vi "Run Action_Do.vi"(8 "error in (no error)":errorcluster, 11 "Set Version from Git Tag":refnum<class "Set Version from Git Tag.lvclass">) -> (0 "error out":errorcluster, 1 "Success?":bool, 3 "Report Array":refnum<class "Report Data.lvclass">[](array[class]))   [LabVIEW 2020, in "ProjectBuilder.lvlib" / "Set Version from Git Tag.lvclass"]
uses:
  Set Version from Git Tag.lvclass
  Action/Project Action/Project Action.lvclass
  ProjectBuilder.lvlib
  <vilib>/AppBuilder/AB_API_Simple/Build Specification Version.ctl
  <vilib>/AppBuilder/AB_API_Simple/NI_App_Builder_API.lvlib
  Version Data/Version Data.lvclass
  C:/Current projects/WS/LV32.2020..ProjectBuilder/Class/Action/Project Action/Project Action.lvclass
  C:/Current projects/WS/LV32.2020..ProjectBuilder/Interface/Project Action Interface/Project Action Interface.lvclass
  C:/Current projects/WS/LV32.2020..ProjectBuilder/Class/Set Version from Git Tag/Set Version from Git Tag.lvclass
  C:/Current projects/WS/LV32.2020..ProjectBuilder/Class/Data/Report Data/Report Data.lvclass
  C:/Current projects/WS/LV32.2020..ProjectBuilder/Class/Set Version from Git Tag/Version Data/Version Data.lvclass
  Data/Report Data/Report Data.lvclass
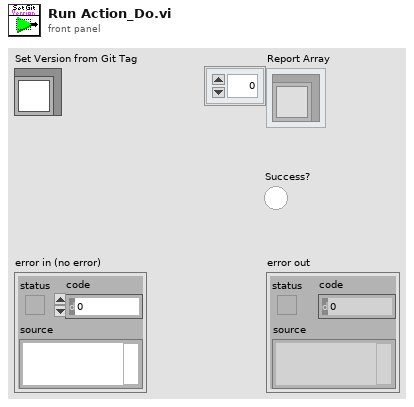
[diagram p1: front panel]
types:
  T1 = typedef "NI_App_Builder_API.lvlib/Build Specification Version.ctl" = cluster{"Major":u16, "Minor":u16, "Fix":u16, "Build":u16}
  T2 = cluster{"Build Specification Version[0]":i32, "Build Specification Version[1]":i32, "Build Specification Version[2]":i32, "Build Specification Version[3]":i32}
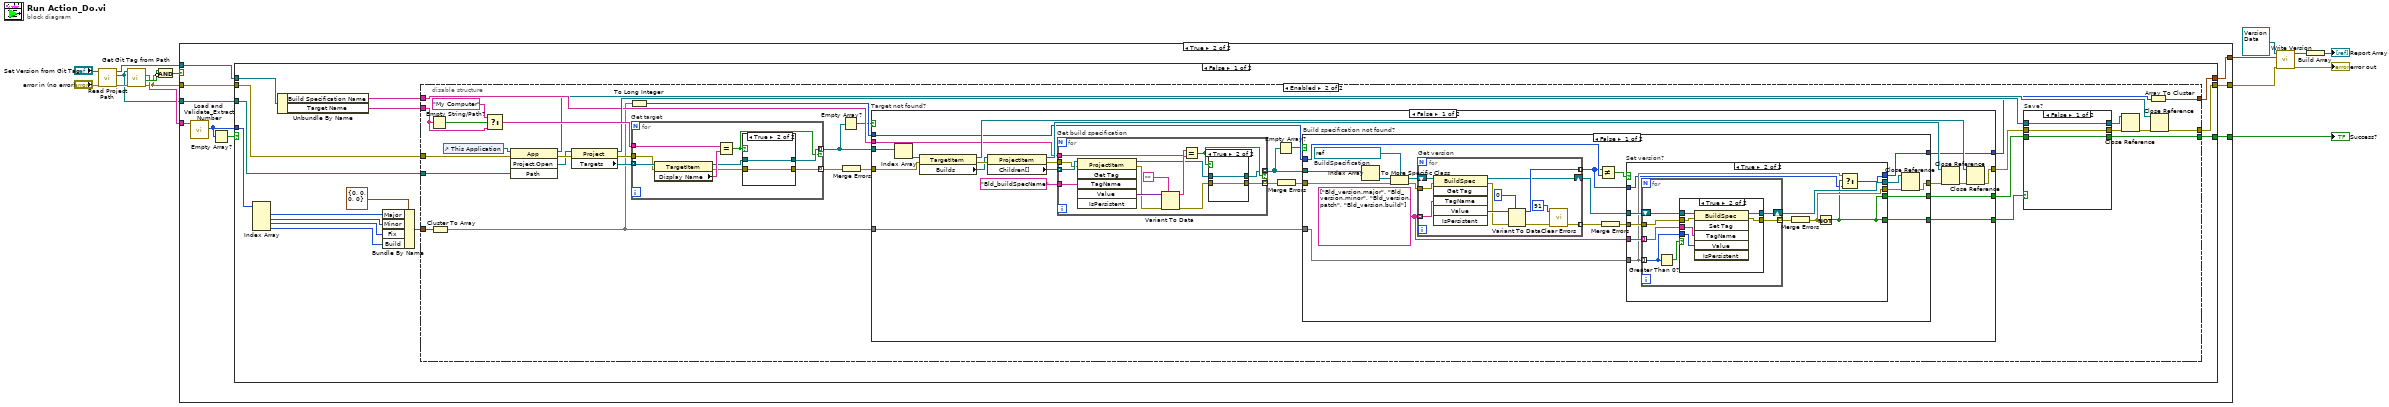
[diagram p0: block diagram]
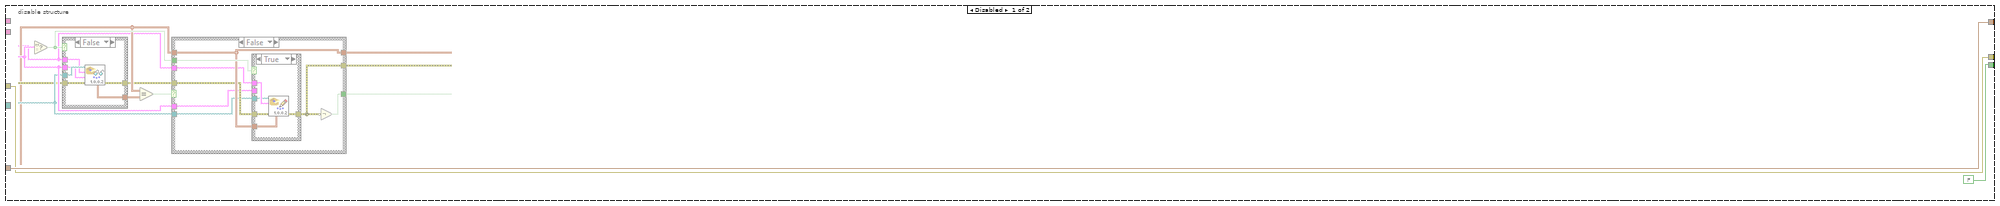
[diagram p3: hidden frame]
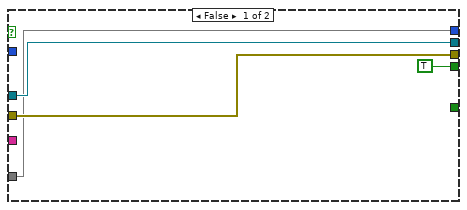
[diagram p4: hidden frame]
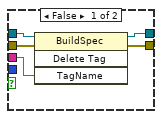
[diagram p5: hidden frame]
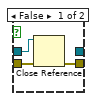
[diagram p7: hidden frame]
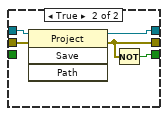
[diagram p9: hidden frame]
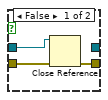
[diagram p10: hidden frame]
diagram:
  n1 = call "Read Project Path.vi"("error in (no error)"="error in (no error)", "Project Action in"="Set Version from Git Tag") -> ("error out"=w14:errorcluster, "Project Path"=w10:path, "Project Action out"=w8:refnum<class "Set Version from Git Tag.lvclass">)  [unwired: 7 in]
  n2 = call "Get Git Tag from Path.vi"("error in (no error)"=w14, "Path"=w10) -> ("error out"=w9:errorcluster, "Success?"=w13:bool, "Tag"=w11:string)  [unwired: 6 in, 1 out]
  n3 = Compound Arithmetic op=AND(w13, invert w9) -> (w12:bool)
  n4 = case shown="True" w12 {
    selector: w12 -> [w17 _]
    tunnel: w11 -> [_ w27]
    tunnel: w10 -> [_ w26]
    tunnel: [w18 w23] -> w7
    tunnel: w9 -> [w18 w24]
    tunnel: [w17 w22] -> w6
    tunnel: w8 -> [_ w25]
    tunnel: [_ w19] -> w1
    frame False {
    }
    frame True {
      n5 = call "Load and Validate_Extract Number.vi"("String"=w27) -> ("Number Array"=w21:i32[])  [unwired: 9 in, 1 out]
      n6 = Empty Array?(array=w21) -> (empty?=w20:bool)
      n7 = case shown="False" w20 {
        tunnel: w26 -> [w29 _]
        tunnel: w25 -> [w37 _]
        tunnel: w24 -> [w30 w205]
        tunnel: [w28 w205] -> w23
        tunnel: [w36 _] -> w22
        tunnel: w21 -> [w35 _]
        tunnel: [w32 _] -> w19
        frame False {
          n8 = Index Array(array=w35) -> (element #1=w41:i32, element #2=w40:i32, element #3=w39:i32, element #4=w38:i32)  [unwired: 4 in]
          n9 = Unbundle By Name(w37) -> ("Build Specification Name"=w34:string, "Target Name"=w31:string)
          n10 = Bundle By Name(cluster=T1 {"Major"=0, "Minor"=0, "Fix"=0, "Build"=0} ("Build Specification Version"), "Major"=w41, "Minor"=w40, "Fix"=w39, "Build"=w38) -> (w33:T1)
          n11 = disable-structure shown="Enabled" {
            disable-tunnel: [FALSE w51] -> w36
            disable-tunnel: w34 -> [_ w62]
            disable-tunnel: w33 -> [w45 w61]
            disable-tunnel: [w45 w48] -> w32
            disable-tunnel: w31 -> [_ w63]
            disable-tunnel: w30 -> [w44 w57]
            disable-tunnel: w29 -> [_ w56]
            disable-tunnel: [w44 w53] -> w28
            frame Disabled {
            }
            frame Enabled {
              n12 = Empty String/Path?(string/path=w63) -> (empty?=w71:bool)
              n13 = Cluster To Array(cluster=w61) -> (array=w60:u16[])
              n14 = control-ref of="This Application"() -> (w55:refnum<vi>)
              n15 = Select(t="My Computer", s=w71, f=w63) -> (s? t:f=w72:string)
              n16 = invoke class="App" method="Project.Open"(reference=w55, error in=w57, "Path"=w56) -> (reference out=w52:refnum<vi>, error out=w70:errorcluster, "Project:Open"=w65:refnum<vi>)  [unwired: 1 in, 1 out]
              n17 = property class="Project"(reference=w65, error in=w70) -> (reference out=w67:refnum<vi>, error out=w75:errorcluster, "Targets"=w73:refnum<vi>[])
              n18 = To Long Integer(number=w60) -> (32bit integer=w59:i32[])
              n19 = for "Get target" {
                tunnel: w73 -> [w199] mode=indexing
                tunnel: w72 -> [w197]
                tunnel: [w195] -> w47 mode=indexing if=w191
                tunnel: w75 -> [w194]
                tunnel: [w192] -> w74 mode=indexing
                n20 = property class="TargetItem"(reference=w199, error in=w194) -> (reference out=w196:refnum<vi>, error out=w193:errorcluster, "Display Name"=w198:string)
                n21 = Equal?(x=w197, y=w198) -> (x = y?=w191:bool)
                n22 = case shown="True" w191 {
                  tunnel: [_ w204] -> w195
                  tunnel: w196 -> [w202 w204]
                  tunnel: w193 -> [w201 w203]
                  tunnel: [w200 w203] -> w192
                  frame False {
                    n23 = Close Reference(reference=w202, error in (no error)=w201) -> (error out=w200:errorcluster)
                  }
                  frame True {
                  }
                }
              }
              n24 = Empty Array?(array=w47) -> (empty?=w46:bool)
              n25 = Merge Errors(w74) -> (w76:errorcluster)
              n26 = case "Target not found?" shown="False" w46 {
                tunnel: w76 -> [w99 w182]
                tunnel: w47 -> [w97 _]
                tunnel: [w91 w182] -> w66
                tunnel: w62 -> [w84 _]
                tunnel: w60 -> [w83 _]
                tunnel: w59 -> [w82 _]
                tunnel: [w81 _] -> w58
                tunnel: [w80 _] -> w50
                tunnel: [w79 _] -> w49
                frame False {
                  n27 = Index Array(array=w97) -> (element=w86:refnum<vi>)  [unwired: 1 in]
                  n28 = property class="TargetItem"(reference=w86, error in=w99) -> (reference out=w98:refnum<vi>, error out=w92:errorcluster, "Builds"=w87:refnum<vi>)
                  n29 = property class="ProjectItem"(reference=w87, error in=w92) -> (reference out=w90:refnum<vi>, error out=w95:errorcluster, "Children[]"=w93:refnum<vi>[])
                  n30 = for "Get build specification" {
                    tunnel: w93 -> [w176] mode=indexing
                    tunnel: "Bld_buildSpecName" ("String") -> [w175]
                    tunnel: w84 -> [w171]
                    tunnel: w95 -> [w170]
                    tunnel: [w167] -> w78 mode=indexing if=w169
                    tunnel: [w164] -> w94 mode=indexing
                    n31 = invoke class="ProjectItem" method="Get Tag"(reference=w176, error in=w170, "TagName"=w175) -> (reference out=w168:refnum<vi>, error out=w166:errorcluster, "Value"=w174:variant)  [unwired: 3 in, 3 out]
                    n32 = Variant To Data(error in=w166, type="", Variant=w174) -> (data=w172:string, error out=w165:errorcluster)
                    n33 = Equal?(x=w171, y=w172) -> (x = y?=w169:bool)
                    n34 = case shown="True" w169 {
                      tunnel: [_ w181] -> w167
                      tunnel: w168 -> [w179 w181]
                      tunnel: w165 -> [w178 w180]
                      tunnel: [w177 w180] -> w164
                      frame False {
                        n35 = Close Reference(reference=w179, error in (no error)=w178) -> (error out=w177:errorcluster)
                      }
                      frame True {
                      }
                    }
                  }
                  n36 = Empty Array?(array=w78) -> (empty?=w77:bool)
                  n37 = Merge Errors(w94) -> (w96:errorcluster)
                  n38 = case "Build specification not found?" shown="False" w77 {
                    tunnel: w96 -> [w118 w163]
                    tunnel: w78 -> [w117 _]
                    tunnel: [w111 w163] -> w88
                    tunnel: w83 -> [w106 _]
                    tunnel: w82 -> [w104 _]
                    tunnel: [w103 _] -> w81
                    tunnel: [w102 _] -> w80
                    tunnel: [w100 _] -> w79
                    frame False {
                      w108 = string[] ["Bld_version.major", "Bld_version.minor", "Bld_version.patch", "Bld_version.build"]
                      w107 = refnum<vi> refnum  # BuildSpecification
                      n39 = Index Array(array=w117) -> (element=w109:refnum<vi>)  [unwired: 1 in]
                      n40 = To More Specific Class(target class=w107, reference=w109, error in=w118) -> (specific class reference=w116:refnum<vi>, error out=w115:errorcluster)
                      n41 = for "Get version" {
                        tunnel: w108 -> [w161] mode=indexing
                        tunnel: [w158] -> w101 mode=indexing
                        shift-right: [w157] -> w110
                        shift-left: w116 -> [w162]
                        tunnel: [w153] -> w113 mode=indexing
                        tunnel: w115 -> [w154]
                        n42 = invoke class="BuildSpec" method="Get Tag"(reference=w162, error in=w154, "TagName"=w161) -> (reference out=w157:refnum<vi>, error out=w156:errorcluster, "Value"=w160:variant)  [unwired: 3 in, 3 out]
                        n43 = Variant To Data(error in=w156, type=0, Variant=w160) -> (data=w158:i32, error out=w155:errorcluster)
                        n44 = call <vilib>:"Clear Errors.vi"("error in (no error)"=w155, "specific error code to clear (0: all)"=91) -> ("error out"=w153:errorcluster)  [unwired: 4 in, 1 out]
                      }
                      n45 = Not Equal?(x=w101, y=w104) -> (x != y?=w105:bool)
                      n46 = Merge Errors(w113) -> (w114:errorcluster)
                      n47 = case "Set version?" shown="True" w105 {
                        tunnel: [w123 w133] -> w119
                        tunnel: w114 -> [w122 w132]
                        tunnel: [w122 w128] -> w112
                        tunnel: w110 -> [w123 w130]
                        tunnel: w108 -> [_ w129]
                        tunnel: w106 -> [w120 w126]
                        tunnel: [_ w127] -> w103
                        tunnel: [TRUE w127] -> w102
                        tunnel: w101 -> [_ w125]
                        tunnel: [w120 w124] -> w100
                        frame False {
                        }
                        frame True {
                          n48 = for {
                            tunnel: w129 -> [w139] mode=indexing
                            shift-right: [w138] -> w133
                            shift-left: w130 -> [w140]
                            tunnel: w126 -> [w135] mode=indexing
                            tunnel: [w137] -> w131 mode=indexing
                            tunnel: w132 -> [w136]
                            n49 = Greater Than 0?(x=w135) -> (x > 0?=w134:bool)
                            n50 = case shown="True" w134 {
                              tunnel: w140 -> [w145 w151]
                              tunnel: w139 -> [w144 w150]
                              tunnel: [w143 w149] -> w138
                              tunnel: [w141 w148] -> w137
                              tunnel: w136 -> [w142 w147]
                              tunnel: w135 -> [_ w146]
                              frame False {
                                n51 = invoke class="BuildSpec" method="Delete Tag"(reference=w145, error in=w142, "TagName"=w144) -> (reference out=w143:refnum<vi>, error out=w141:errorcluster)  [unwired: 1 in, 2 out]
                              }
                              frame True {
                                n52 = invoke class="BuildSpec" method="Set Tag"(reference=w151, error in=w147, "TagName"=w150, "Value"=w146) -> (reference out=w149:refnum<vi>, error out=w148:errorcluster)  [unwired: 2 in, 4 out]
                              }
                            }
                          }
                          n53 = Merge Errors(w131) -> (w128:errorcluster)
                          n54 = Not(x=w128) -> (.not. x?=w127:bool)
                          n55 = Select(t=w126, s=w127, f=w125) -> (s? t:f=w124:i32[])
                        }
                      }
                      n56 = Close Reference(reference=w119, error in (no error)=w112) -> (error out=w111:errorcluster)
                    }
                    frame True {
                    }
                  }
                  n57 = Close Reference(reference=w90, error in (no error)=w88) -> (error out=w89:errorcluster)
                  n58 = Close Reference(reference=w98, error in (no error)=w89) -> (error out=w91:errorcluster)
                }
                frame True {
                }
              }
              n59 = case "Save?" shown="False" w58 {
                tunnel: [w184 w186] -> w69
                tunnel: [w185 w190] -> w68
                tunnel: w67 -> [w185 w189]
                tunnel: w66 -> [w184 w188]
                tunnel: [w183 w187] -> w51
                tunnel: w50 -> [w183 _]
                frame False {
                }
                frame True {
                  n60 = invoke class="Project" method="Save"(reference=w189, error in=w188) -> (reference out=w190:refnum<vi>, error out=w186:errorcluster)  [unwired: 2 in, 2 out]
                  n61 = Not(x=w186) -> (.not. x?=w187:bool)
                }
              }
              n62 = Close Reference(reference=w68, error in (no error)=w69) -> (error out=w54:errorcluster)
              n63 = Array To Cluster(array=w49) -> (cluster=w48:T2)
              n64 = Close Reference(reference=w52, error in (no error)=w54) -> (error out=w53:errorcluster)
            }
          }
        }
        frame True {
        }
      }
    }
  }
  "Success?" <- w6
  n65 = call "Write Version.vi"("error in (no error)"=w7, "Build Specification Version"=w1, "Version Data in"=refnum<class "Version Data.lvclass"> refnum ("ProjectBuilder.lvlib:Version Data.lvclass")) -> ("error out"=→"error out":errorcluster, "Version Data out"=w2:refnum<class "Version Data.lvclass">)  [unwired: 7 in]
  n66 = Build Array(w2) -> (→"Report Array":refnum<class "Version Data.lvclass">[])
